vi "Example - Simple.vi"() -> ()   [LabVIEW 2017]
uses:
  DO_class/DO.lvclass
panel:
  in  "DO Status to Set":bool
  in  "DO Channel Number (Zero Based)":i32
  out "DO Channel Status":bool
  in  "Quit Program":bool
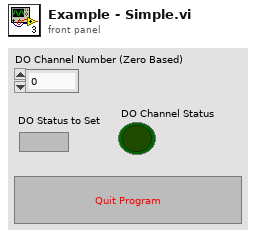
[diagram p1: front panel]
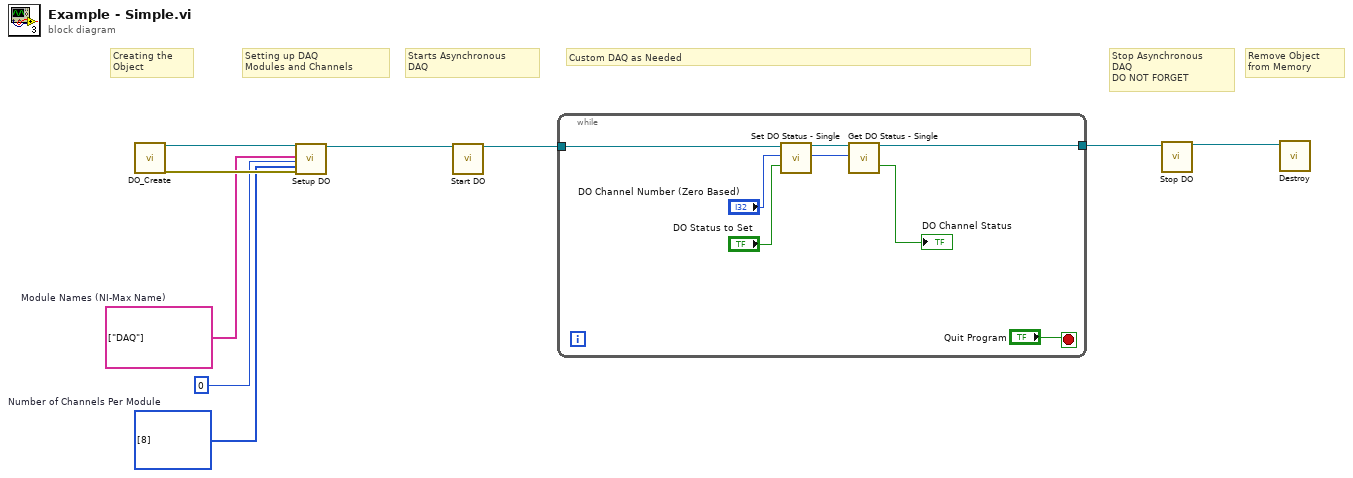
[diagram p0: block diagram]
diagram:
  w7 = u32[] [8]  # Number of Channels Per Module
  w2 = string[] ["DAQ"]  # Module Names (NI-Max Name)
  # "Creating the\nObject"
  # "Setting up DAQ\nModules and Channels"
  # "Custom DAQ as Needed"
  # "Remove Object\nfrom Memory"
  # "Stop Asynchronous\nDAQ\nDO NOT FORGET"
  # "Starts Asynchronous\nDAQ"
  n1 = call "DO_Create.vi"() -> ("reference out"=w9:refnum<class "DO.lvclass">, "error out"=w8:errorcluster)  [unwired: 18 in]
  n2 = call "Setup DO.vi"("reference in"=w9, "Module Names (NI-MAX Alias)"=w2, "DAQ Port Number"=u32 0, "Number of Channels Per Module"=w7, "error in (no error)"=w8) -> ("reference out"=w6:refnum<class "DO.lvclass">)  [unwired: 10 in, 4 out]
  n3 = call-dynamic "Start DO.vi"("reference in"=w6) -> ("reference out"=w4:refnum<class "DO.lvclass">)  [unwired: 17 in, 1 out]
  n4 = while {
    tunnel: w4 -> [w16]
    tunnel: [w14] -> w3
    stop <- "Quit Program" stop-if-true
    n5 = call-dynamic "Set DO Status - Single.vi"("reference in"=w16, "DO Channel Number (Zero Based)"="DO Channel Number (Zero Based)", "DO Status to Set"="DO Status to Set") -> ("reference out"=w15:refnum<class "DO.lvclass">, "DO Channel Number (Zero Based) OUT"=w13:i32)  [unwired: 14 in, 1 out]
    n6 = call-dynamic "Get DO Status - Single.vi"("reference in"=w15, "DO Channel Number (Zero Based)"=w13) -> ("reference out"=w14:refnum<class "DO.lvclass">, "DO Channel Status"=→"DO Channel Status":bool)  [unwired: 15 in, 1 out]
  }
  n7 = call-dynamic "Stop DO.vi"("reference in"=w3) -> ("reference out"=w5:refnum<class "DO.lvclass">)  [unwired: 17 in, 1 out]
  n8 = call-dynamic "Destroy.vi"("reference in"=w5) -> ()  [unwired: 17 in, 2 out]
